vi "SetGain.vi"(8 "error in (no error)":errorcluster, 10 "Arg":string, 11 "PCO in":refnum<class "PCO_Camera.lvclass">) -> (0 "error out":errorcluster, 2 "setValue out":dbl, 3 "PCO out":refnum<class "PCO_Camera.lvclass">)   [LabVIEW 2020, in "PCO_Camera.lvclass"]
uses:
  PCO_Camera.lvclass
  PCO_Camera.lvclass/PCO_Camera.ctl
  Camera.lvclass
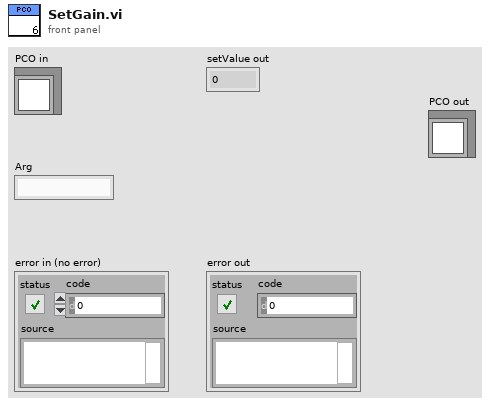
[diagram p1: front panel]
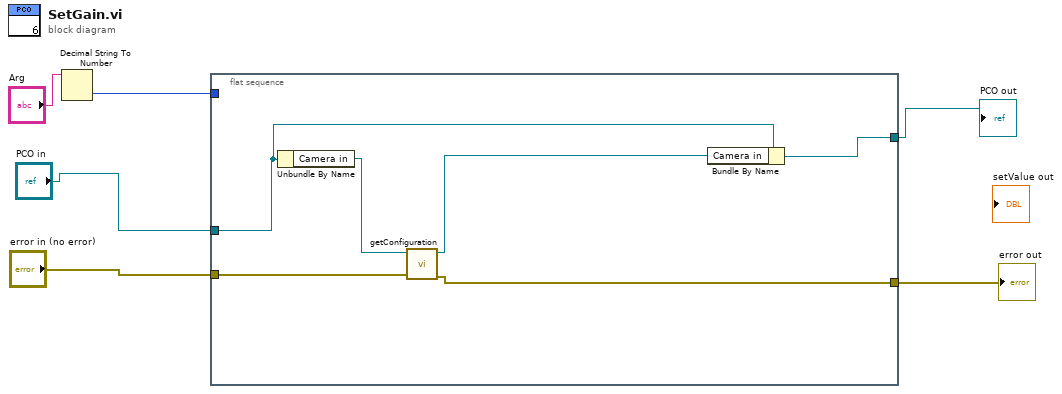
[diagram p0: block diagram]
diagram:
  n1 = Decimal String To Number(string="Arg") -> (number=w2:i32)  [unwired: 2 in, 1 out]
  n2 = flat-sequence {
    tunnel: [w12] -> w4
    tunnel: "error in (no error)" -> [w11]
    tunnel: w2 -> [_]
    tunnel: "PCO in" -> [w10]
    tunnel: [w7] -> w1
    frame #0 {
      n3 = Unbundle By Name(w10) -> ("Camera in"=w9:refnum<class "Camera.lvclass">)
      n4 = call-dynamic "getConfiguration.vi"("error in (no error)"=w11, "Camera in"=w9) -> ("error out"=w7:errorcluster, "Camera out"=w8:refnum<class "Camera.lvclass">)  [unwired: 7 in, 1 out]
      n5 = Bundle By Name(cluster=w10, "Camera in"=w8) -> (w12:refnum<class "PCO_Camera.lvclass">)
    }
  }
  "PCO out" <- w4
  "error out" <- w1
